vi "Process.vi"(8 "error in":errorcluster, 11 "instrument.PPMS":refnum<class "instrument.PPMS.lvclass">) -> (0 "error out":errorcluster, 3 "instrument.PPMS out":refnum<class "instrument.PPMS.lvclass">)   [LabVIEW 2019, in "instrument.PPMS.lvclass"]
doc: "---------------------------------------------------------------\nJKI State Machine Objects™\nhttp://jki.net/state-machine-objects/\nCopyright (C) 2005-2015, JKI <info@jki.net>\nALL RIGHTS RESERVED"
uses:
  instrument.PPMS.lvclass
  <vilib>/JKI/JKI SMO/SMO/SMO.lvclass
  <userlib>/LevyLab/Instrument Framework/Instrument Types/Cryostat/Instrument.Cryostat.lvclass
  <userlib>/LevyLab/RemoteControl/RemoteControl/Typedefs/Message--Cluster.ctl
  <userlib>/LevyLab/RemoteControl/RemoteControl/RemoteControl.lvclass
  Typedefs/Private Events--MessageToProcess.ctl
  <userlib>/LevyLab/Instrument Framework/Instrument/Instrument.lvclass
  <userlib>/LevyLab/Debug/Debug.lvlib
  C:/Program Files (x86)/National Instruments/LabVIEW 2019/user.lib/LevyLab/Instrument Framework/Instrument Types/Cryostat/Instrument.Cryostat.lvclass
  C:/Program Files (x86)/National Instruments/LabVIEW 2019/user.lib/LevyLab/Instrument Framework/Instrument/Instrument.lvclass
  C:/Program Files (x86)/National Instruments/LabVIEW 2019/vi.lib/JKI/JKI SMO/SMO/SMO.lvclass
panel:
  out "Log Address":string
  out "Log Data":variant
  out "Commands":string
  out "Status":string
  in  "STOP":bool
  # "PPMS Monitor"
  # "THIS ONE IS NOT THE UI"
  # "For instructions on how to use the JKI State Machine Objects, examples and video tutorials, visit:\nhttp://jki.net/state-machine-objects/\n\nJKI State Machine Objects™\nhttp://jki.net/state-machine-objects/\nCopyright (C) 2005-2015, JKI <info@jki.net>\nALL RIGHTS RESERVED"
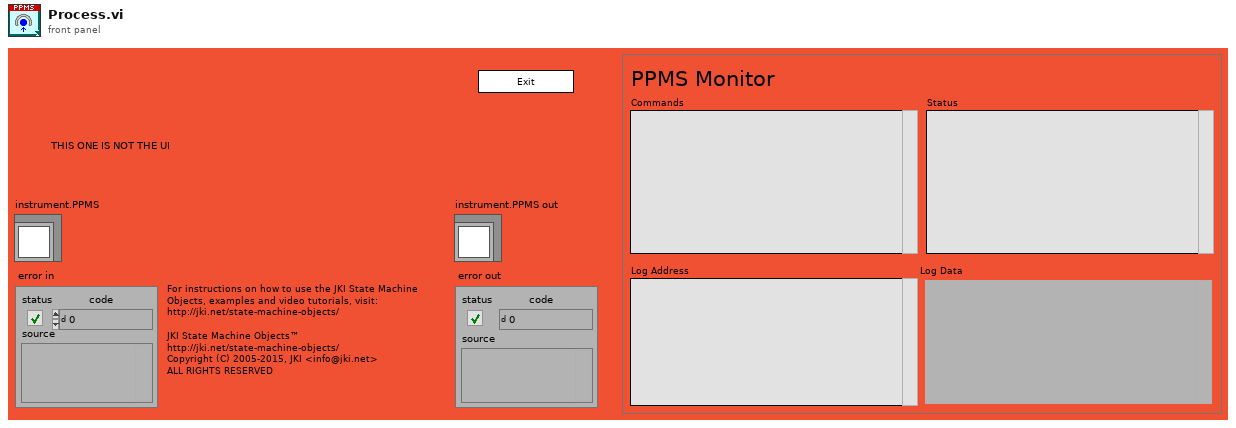
[diagram p1: front panel]
types:
  T1 = enum32{"invalid app kind", "Development System", "Run Time System", "Student Edition", "Embedded LabVIEW", "Evaluation", "Custom"}
  T2 = enum32{"Invalid", "Standard", "Closed", "Hidden", "Minimized", "Maximized"}
  T3 = typedef "RemoteControl.lvlib/RemoteControl.lvclass/Message--Cluster.ctl" = cluster{"Command":string, "Data":variant, "ID":string, "error":errorcluster}
  T4 = typedef "instrument.PPMS.lvclass/Private Events--MessageToProcess.ctl" = cluster{"Message":T3}
  T5 = cluster{"Core":cluster{"Current VI Reference":refnum<vi>, "Close Panel on Exit?":bool, "Last Error":cluster{"error":errorcluster, "previous state":string, "remaining states":string}, "Shutdown?":bool}, "SMO":refnum<class "instrument.PPMS.lvclass">, "MessageToProcess":T4}
  T6 = cluster{"Current VI Reference":refnum<vi>, "Close Panel on Exit?":bool, "Last Error":cluster{"error":errorcluster, "previous state":string, "remaining states":string}, "Shutdown?":bool}
  T7 = typedef "instrument.PPMS.lvclass/PPMS.getAll--cluster.ctl" = cluster{"Chamber Status":string, "Helium Level":dbl, "Temperature":dbl, "Temperature Status":string, "Magnetic Field":dbl, "Magnet Status":string, "Position":dbl}
  T8 = typedef "Debug.lvlib/Attribute.Debug.lvclass/DebugBehavior.ctl" = enum16{"Normal", "Debug"}
  T9 = typedef "SMO.lvclass/Protected Events.ctl" = cluster{"StopProcesses":refnum<user-event>, "AbortProcesses":refnum<user-event>, "Config Changed":refnum<user-event>, "Dependency":refnum<user-event>}
  T10 = typedef "instrument.PPMS.lvclass/Private Events--Cluster.ctl" = cluster{"MessageToProcess":refnum<user-event>}
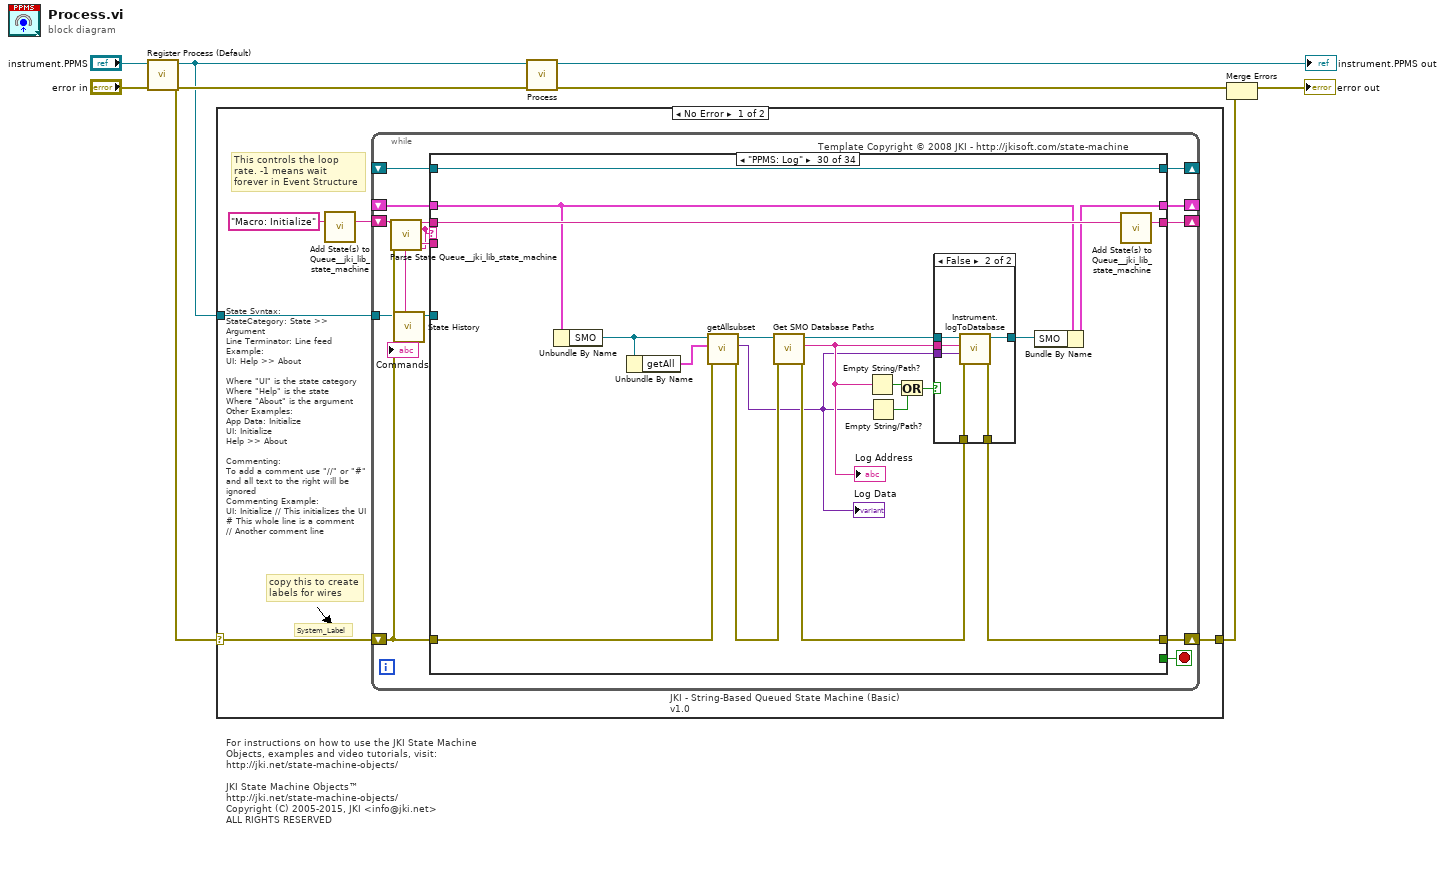
[diagram p0: block diagram]
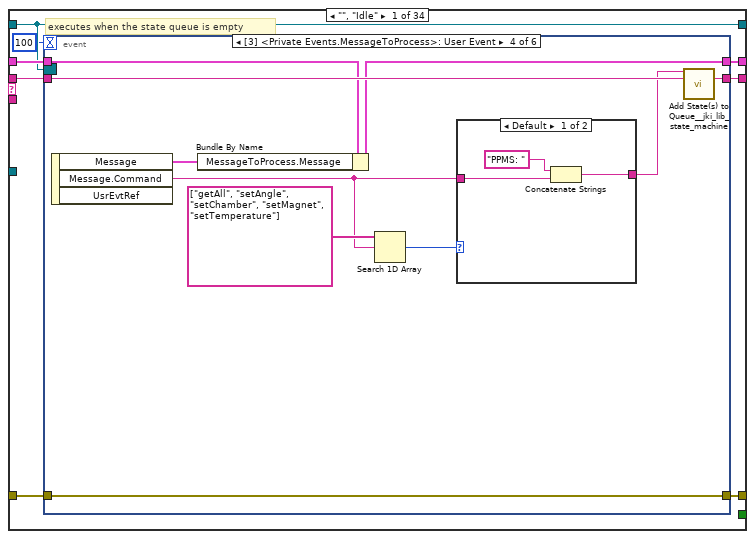
[diagram p2: hidden frame]
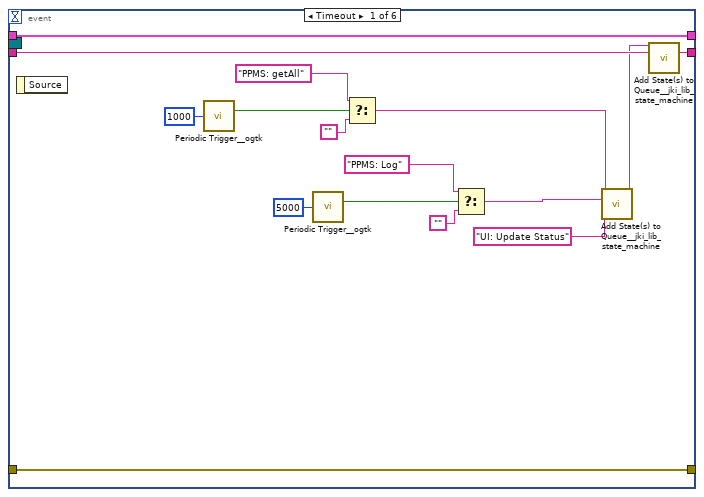
[diagram p3: hidden frame]
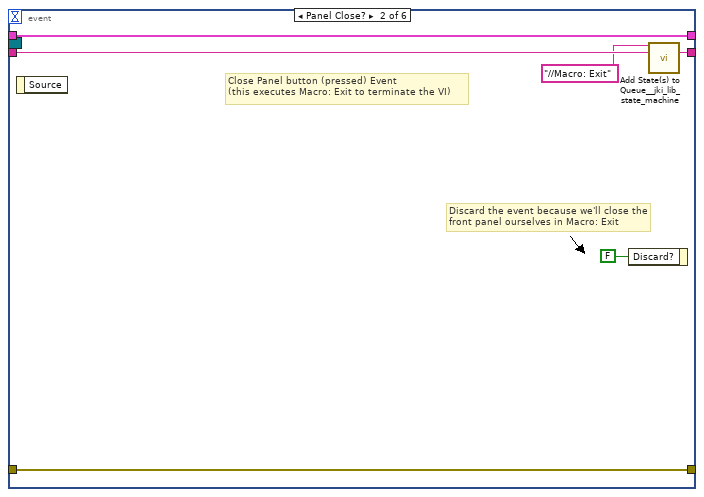
[diagram p4: hidden frame]
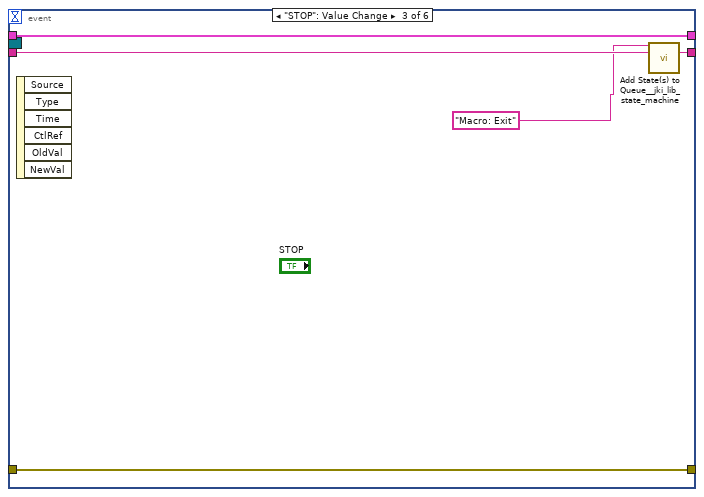
[diagram p5: hidden frame]
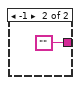
[diagram p6: hidden frame]
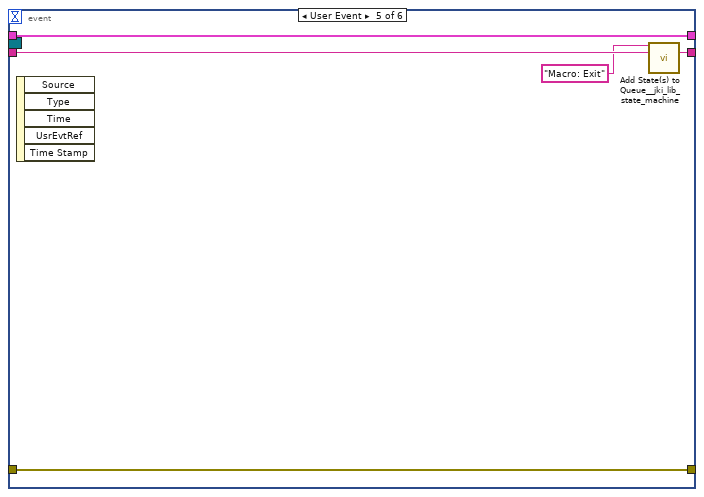
[diagram p7: hidden frame]
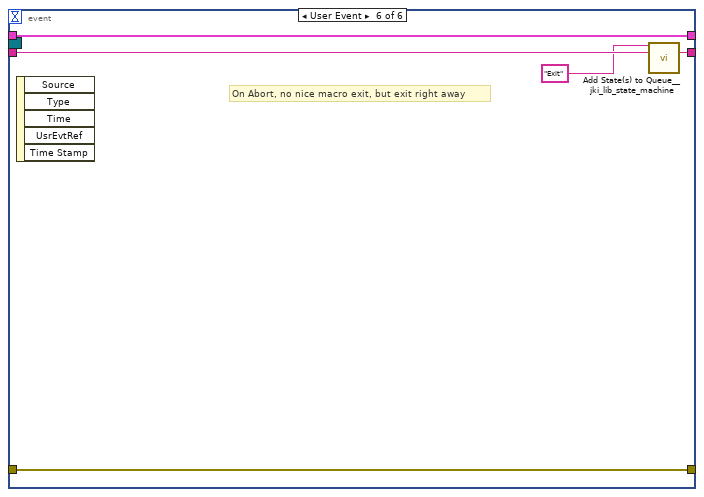
[diagram p8: hidden frame]
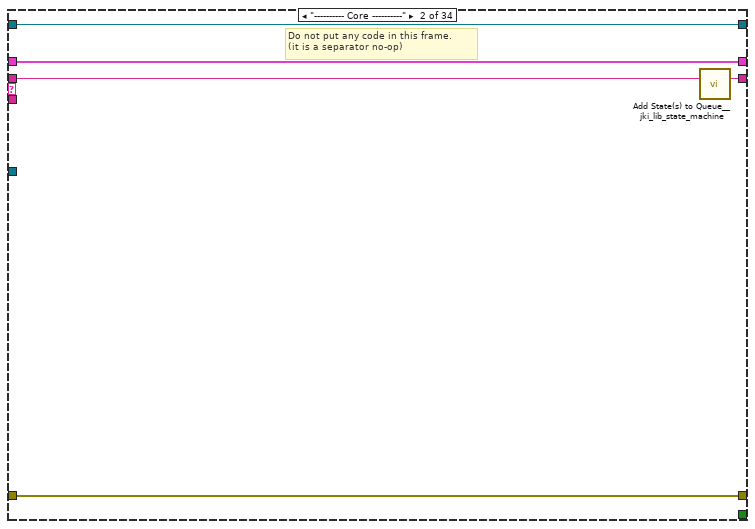
[diagram p9: hidden frame]
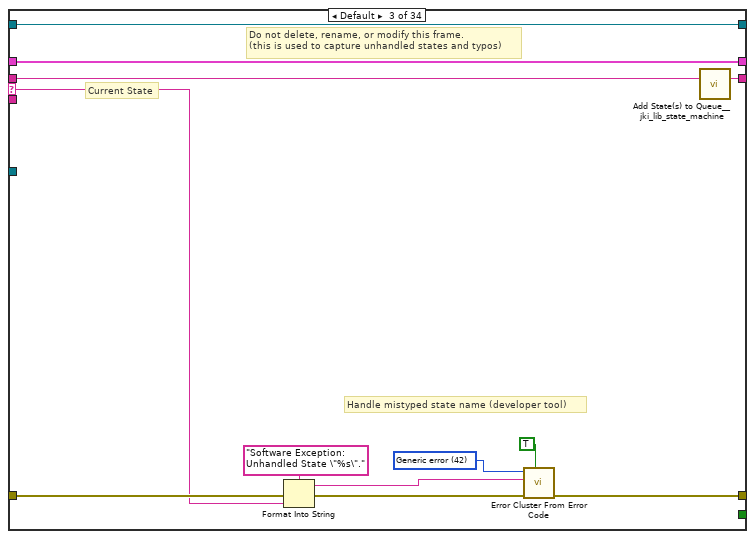
[diagram p10: hidden frame]
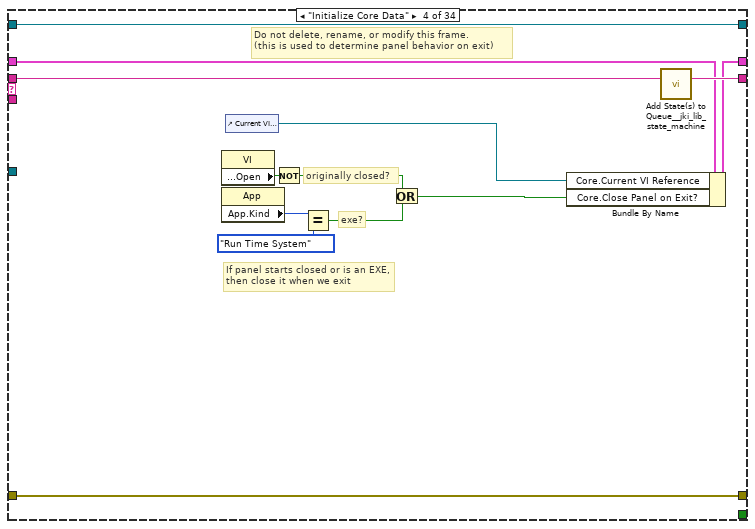
[diagram p11: hidden frame]
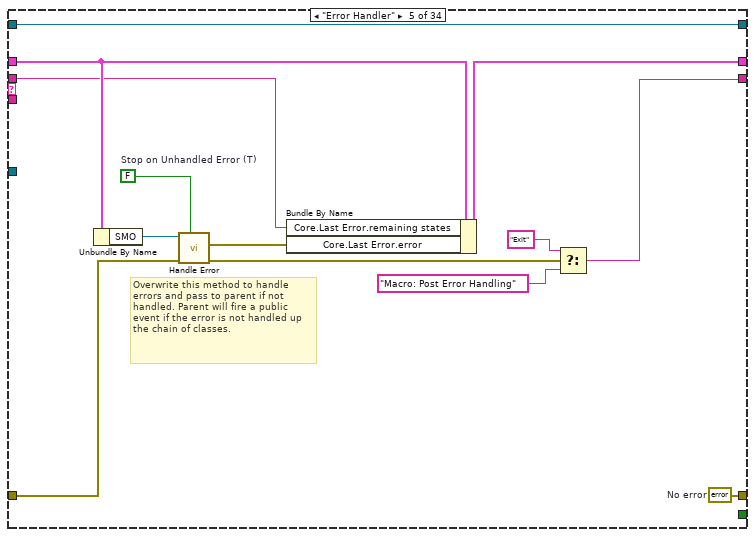
[diagram p12: hidden frame]
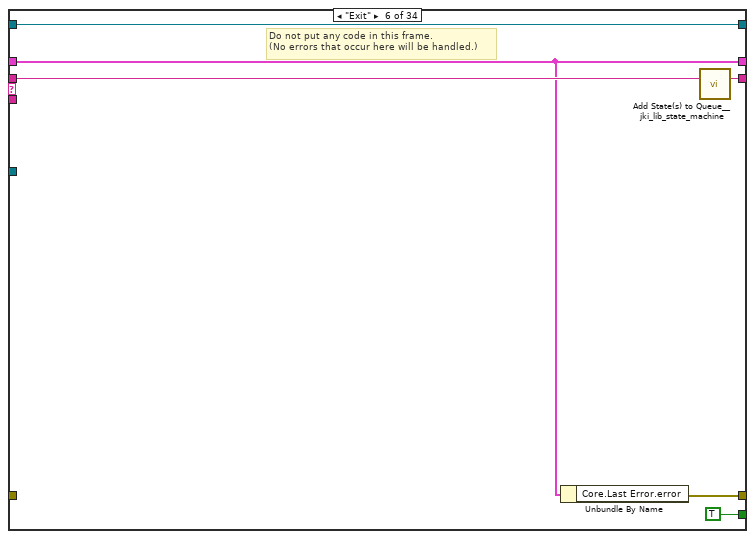
[diagram p13: hidden frame]
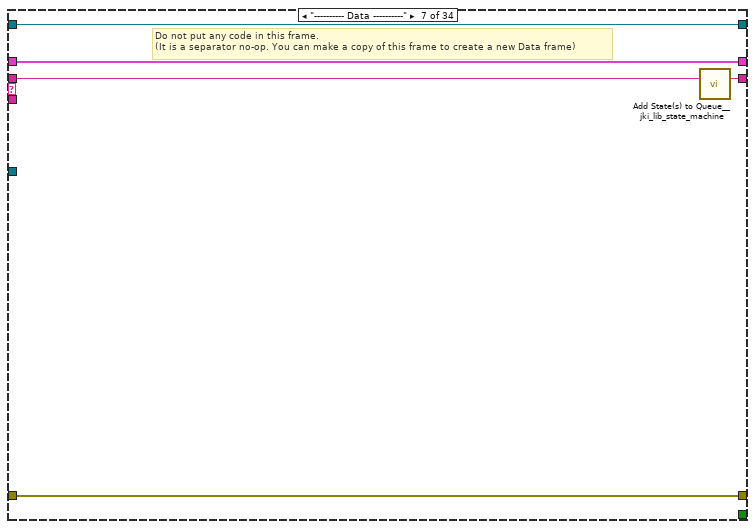
[diagram p14: hidden frame]
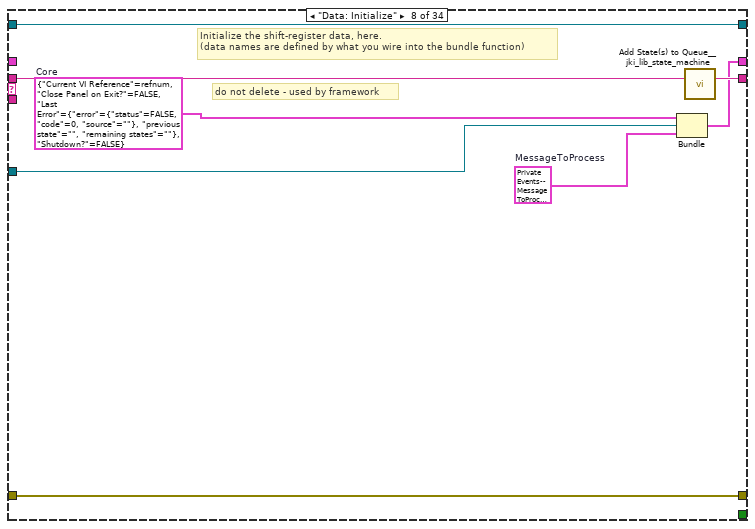
[diagram p15: hidden frame]
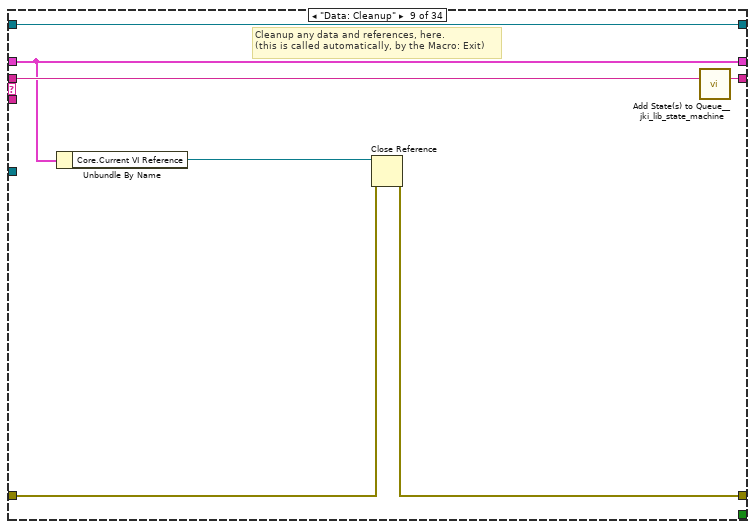
[diagram p16: hidden frame]
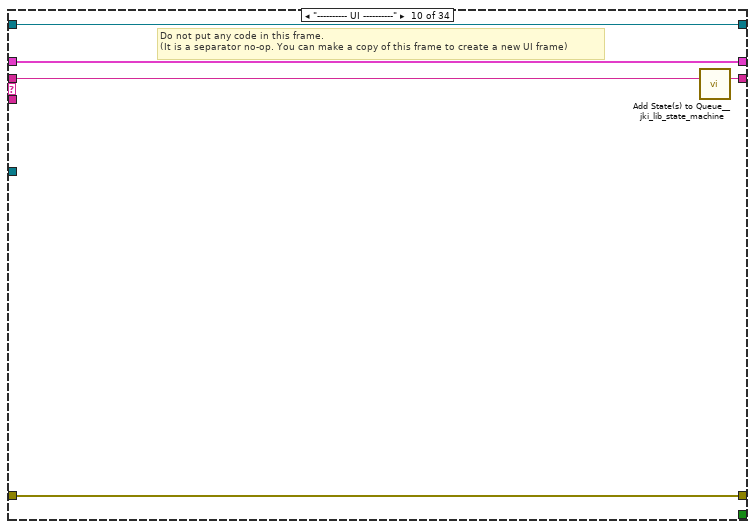
[diagram p17: hidden frame]
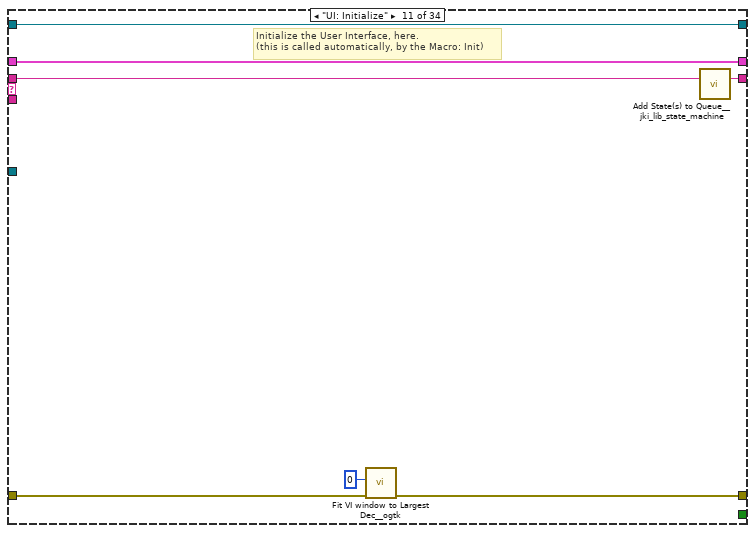
[diagram p18: hidden frame]
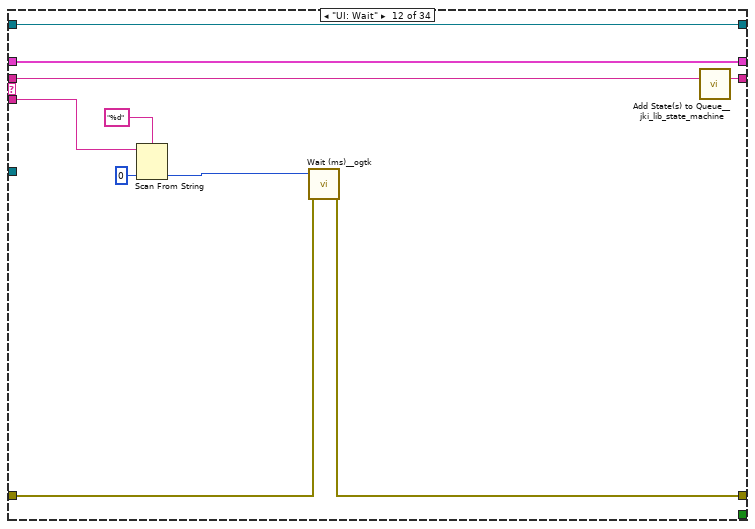
[diagram p19: hidden frame]
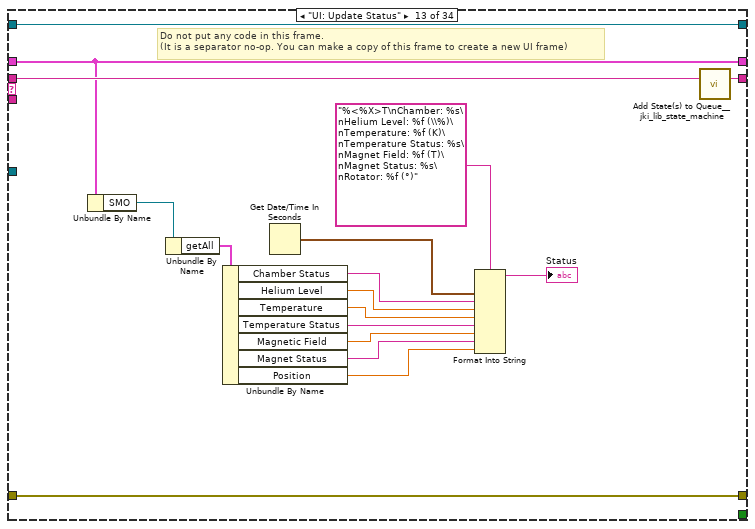
[diagram p20: hidden frame]
diagram:
  # "For instructions on how to use the JKI State Machine Objects, examples and video tutorials, visit:\nhttp://jki.net/state-machine-objects/\n\nJKI State Machine Objects™\nhttp://jki.net/state-machine-objects/\nCopyright (C) 2005-2015, JKI <info@jki.net>\nALL RIGHTS RESERVED"
  n1 = call <vilib>:"Register Process (Default).vi"("error in (no error)"="error in", "SMO"="instrument.PPMS") -> ("error out"=w5:errorcluster, "SelfRef"=w4:refnum<class "instrument.PPMS.lvclass">)  [unwired: 8 in]
  n2 = case shown="No Error" w5 {
    selector: w5 -> [w10 w454]
    tunnel: w4 -> [w11 _]
    tunnel: [w9 w454] -> w1
    frame No Error {
      # "State Syntax:\nStateCategory: State >> Argument\nLine Terminator: Line feed\nExample:\nUI: Help >> About\n\nWhere \"UI\" is the state category\nWhere \"Help\" is the state\nWhere \"About\" is the argument\nOther Examples:\nApp Data: Initialize\nUI: Initialize\nHelp >> About\n\nCommenting:\nTo add a comment use \"//\" or \"#\" and all text to the right will be ignored\nCommenting Example:\nUI: Initialize // This initializes the UI\n# This whole line is a comment\n// Another comment line"
      # "copy this to create labels for wires"
      # "This controls the loop rate. -1 means wait forever in Event Structure"
      # "System_Label"
      n3 = call <vilib>:"Add State(s) to Queue__jki_lib_state_machine.vi"("State(s) in (\"\")"="Macro: Initialize") -> ("States Out"=w13:string)  [unwired: 14 in]
      n4 = while "JKI - String-Based Queued State Machine (Basic) v1.0" {
        shift-right: [w23] -> _
        shift-left: _ -> [w19]
        shift-right: [w26] -> w9
        shift-left: w10 -> [w22]
        shift-right: [w25] -> _
        shift-left: w13 -> [w27]
        tunnel: w11 -> [w14]
        shift-right: [w21] -> _
        shift-left: _ -> [w20]
        stop <- w24 stop-if-true
        # "Template Copyright © 2008 JKI - http://jkisoft.com/state-machine"
        n5 = call <vilib>:"Parse State Queue__jki_lib_state_machine.vi"("State Queue"=w27, "Error In (no error)"=w22) -> ("Remaining States"=w28:string, "Current State"=w17:string, "Arguments"=w18:string)  [unwired: 11 in]
        n6 = call <userlib>:"State History.vi"("Current State"=w17, "SMO"=w14) -> ("SMO"=w15:refnum<class "instrument.PPMS.lvclass">, "History"=→"Commands":string)  [unwired: 8 in]
        n7 = case shown="\"PPMS: Log\"" w17 {
          selector: w17 -> [_ _ w94 _ _ _ _ _ _ _ _ _ _ _ _ _ _ _ _ _ _ _ _ _ _ _ _ _ _ _ _ _ _ _]
          tunnel: w28 -> [w36 w92 w98 w117 w118 w136 w141 w149 w156 w161 w168 w178 w195 w202 w218 w250 w259 w273 w290 w311 w316 w327 w332 w345 w351 w356 w365 w374 w386 w405 w423 w433 w443 w453]
          tunnel: w18 -> [_ _ _ _ _ _ _ _ _ _ _ w170 _ w196 w212 _ _ _ _ _ _ _ _ _ _ _ _ _ _ _ _ _ _ _]
          tunnel: w19 -> [w34 w89 w96 w108 w126 w132 w138 _ w152 w158 w166 w175 w182 w200 w214 w247 w255 w261 w280 w295 w313 w324 w329 w343 w349 w353 w361 w370 w380 w400 w419 w429 w439 w449]
          tunnel: [w33 w90 w100 w114 w127 w131 w139 w142 w153 w159 w163 w174 w193 w197 w215 w248 w257 w271 w288 w309 w314 w318 w330 w338 w347 w354 w358 w366 w377 w399 w415 w425 w435 w445] -> w26
          tunnel: w22 -> [w32 w90 w99 w114 w128 _ w139 w142 w150 w159 w162 w173 w193 w198 w216 w248 w257 w271 w288 w309 w314 w319 w330 w339 w347 w354 w359 w367 w382 w392 w416 w426 w436 w446]
          tunnel: [w35 w91 w97 w116 w119 w135 w140 w148 w155 w160 w167 w177 w194 w201 w217 w249 w258 w272 w289 w310 w315 w326 w331 w344 w350 w355 w364 w373 w385 w404 w422 w432 w442 w452] -> w25
          tunnel: [_ _ _ _ _ TRUE _ _ _ _ _ _ _ _ _ _ _ _ _ _ _ _ _ _ _ _ _ _ _ _ _ _ _ _] -> w24
          tunnel: [w31 w89 w96 w115 w125 w132 w138 w146 w152 w158 w166 w175 w182 w200 w214 w247 w255 w262 w281 w296 w313 w324 w329 w343 w349 w353 w362 w371 w381 w401 w420 w430 w440 w450] -> w23
          tunnel: w15 -> [_ _ _ _ _ _ _ w143 _ _ _ _ _ _ _ _ _ _ _ _ _ _ _ _ _ _ _ _ _ _ _ _ _ _]
          tunnel: [w30 w88 w93 w105 w130 w133 w137 w147 w151 w157 w165 w176 w192 w199 w211 w246 w256 w270 w287 w303 w312 w325 w328 w342 w348 w352 w363 w372 w384 w403 w421 w431 w441 w451] -> w21
          tunnel: w20 -> [w30 w88 w93 w105 w130 w133 w137 w147 w151 w157 w165 w176 w192 w199 w211 w246 w256 w270 w287 w303 w312 w325 w328 _ w348 w352 w363 w372 w384 w403 w421 w431 w441 w451]
          frame "", "Idle" {
            # "executes when the state queue is empty"
            n8 = event shown="[3] <Private Events.MessageToProcess>: User Event" {
              selector: w30 -> [_ _ _ _ _ _]
              dyn-events: _ -> [_ _ _ _ _ _]
              timeout: 100 -> [_ _ _ _ _ _]
              tunnel: w36 -> [w52 w58 w63 w73 w82 w87]
              tunnel: [w51 w57 w62 w72 w81 w86] -> w35
              tunnel: w34 -> [w50 w55 w60 w68 w79 w84]
              tunnel: [w49 w56 w61 w71 w80 w85] -> w33
              tunnel: w32 -> [w49 w56 w61 w71 w80 w85]
              tunnel: [w50 w55 w60 w69 w79 w84] -> w31
              event Timeout {
                n9 = event-data() -> ()  [unwired: 1 in, 1 out]
                n10 = call <userlib>:"Periodic Trigger__ogtk.vi"("time (ms)"=u32 1000) -> ("Triggered"=w48:bool)  [unwired: 12 in, 2 out]
                n11 = call <userlib>:"Periodic Trigger__ogtk.vi"("time (ms)"=u32 5000) -> ("Triggered"=w39:bool)  [unwired: 12 in, 2 out]
                n12 = Select(t="PPMS: getAll", s=w48, f="") -> (s? t:f=w43:string)
                n13 = Select(t="PPMS: Log", s=w39, f="") -> (s? t:f=w37:string)
                n14 = call <vilib>:"Add State(s) to Queue__jki_lib_state_machine.vi"("State(s) in Front (\"\")"=w43, "State(s) in (\"\")"=w37, "State(s) at Back (\"\")"="UI: Update Status") -> ("States Out"=w42:string)  [unwired: 12 in]
                n15 = call <vilib>:"Add State(s) to Queue__jki_lib_state_machine.vi"("State(s) in Front (\"\")"=w42, "State(s) in (\"\")"=w52) -> ("States Out"=w51:string)  [unwired: 13 in]
              }
              event Panel Close? {
                # "Discard the event because we'll close the front panel ourselves in Macro: Exit"
                # "Close Panel button (pressed) Event\n(this executes Macro: Exit to terminate the VI)"
                n16 = event-data() -> ()  [unwired: 1 in, 1 out]
                n17 = event-data("Discard?"=FALSE) -> ()  [unwired: 1 in, 1 out]
                n18 = call <vilib>:"Add State(s) to Queue__jki_lib_state_machine.vi"("State(s) in Front (\"\")"="//Macro: Exit", "State(s) in (\"\")"=w58) -> ("States Out"=w57:string)  [unwired: 13 in]
              }
              event "STOP": Value Change {
                n19 = event-data() -> ()  [unwired: 1 in, 6 out]
                n20 = call <vilib>:"Add State(s) to Queue__jki_lib_state_machine.vi"("State(s) in Front (\"\")"="Macro: Exit", "State(s) in (\"\")"=w63) -> ("States Out"=w62:string)  [unwired: 13 in]
              }
              event User Event {
                n21 = event-data() -> ("Message"=w70:T3, "Message.Command"=w64:string)  [unwired: 1 in, 1 out]
                n22 = Bundle By Name(cluster=w68, "MessageToProcess.Message"=w70) -> (w69:T5)
                n23 = Search 1D Array(1D array=string[] ["getAll", "setAngle", "setChamber", "setMagnet", "setTemperature"], element=w64) -> (index of element=w67:i32)  [unwired: 1 in]
                n24 = case shown="Default" w67 {
                  tunnel: [w76 ""] -> w66
                  tunnel: w64 -> [w75 _]
                  frame Default {
                    n25 = Concatenate Strings("PPMS: ", w75) -> (w76:string)
                  }
                  frame -1 {
                  }
                }
                n26 = call <vilib>:"Add State(s) to Queue__jki_lib_state_machine.vi"("State(s) in Front (\"\")"=w66, "State(s) in (\"\")"=w73) -> ("States Out"=w72:string)  [unwired: 13 in]
              }
              event User Event {
                n27 = event-data() -> ()  [unwired: 1 in, 5 out]
                n28 = call <vilib>:"Add State(s) to Queue__jki_lib_state_machine.vi"("State(s) in Front (\"\")"="Macro: Exit", "State(s) in (\"\")"=w82) -> ("States Out"=w81:string)  [unwired: 13 in]
              }
              event User Event {
                # "On Abort, no nice macro exit, but exit right away"
                n29 = event-data() -> ()  [unwired: 1 in, 5 out]
                n30 = call <vilib>:"Add State(s) to Queue__jki_lib_state_machine.vi"("State(s) in Front (\"\")"="Exit", "State(s) in (\"\")"=w87) -> ("States Out"=w86:string)  [unwired: 13 in]
              }
            }
          }
          frame "---------- Core ----------" {
            # "Do not put any code in this frame.\n(it is a separator no-op)"
            n31 = call <vilib>:"Add State(s) to Queue__jki_lib_state_machine.vi"("State(s) in (\"\")"=w92) -> ("States Out"=w91:string)  [unwired: 14 in]
          }
          frame Default {
            w103 = 42 items=["No error", "Argument error", "Memory is full", "Out of zone", "End of file", "File already open", "Generic file I/O error", "File not found", "File permission error", "Disk is full", "Duplicate path", "Too many files open", "System feature not enabled", "Resource file not found", "Cannot add resource", "Resource not found", "Image not found", "Image memory error", "Pen does not exist", "Config type invalid", "Config token not found", "Config parse error", "Config memory error", "Bad external code format", "Bad external code offset", "External code not present", "Null window", "Destroy window error", "Null menu", "Print aborted", "Bad print record", "Print driver error", "Windows error during printing", "Memory error during printing", "Print dialog error", "Generic print error", "Invalid device refnum", "Device not found", "Device parameter error", "Device unit error", "Cannot open device", "Device call aborted", "Generic error", "Cancelled by user", "Object ID too low", "Object ID too high", "Object not in heap", "Unknown heap", "Unknown object (invalid DefProc)", "Unknown object (DefProc not in table)", "Message out of range", "Invalid (null) method", "Unknown message", "Manager call not supported", "Bad address", "Network operation in progress", "Network operation timed out", "Connection is busy", "Network attribute not supported", "Network error", "Address in use", "System out of memory", "Connection aborted", "Connection refused", "Not connected", "Already connected", "Connection closed", "Initialization error (interapplication manager)", "Bad occurrence", "Wait on unbound occurrence handler", "Occurrence queue overflow", "Datalog type conflict", "Unused", "Unrecognized type (interapplication manager)", "Memory corrupt", "Failed to make temporary DLL", "Old CIN version", "Drag socket not found", "Failed to load drop-object", "Failed to register OLE object", "Failed to release OLE object", "Format specifier type mismatch", "Unknown format specifier", "Too few format specifiers", "Too many format specifiers", "Scan failed", "Newer CIN version", "Error converting to variant", "Runtime menu error", "Password tampered", "Variant attribute not found", "Incompatible variant data type", "Event data is not available", "Event Store is not present", "Occurrence is not found", "Event Queue is not created", "Event info is not available", "Refnum passed is NULL", "Error retrieving Class GUID", "Error retrieving CoClass GUID", "Error retrieving TypeLib GUID.", "Bad built application magic bytes.", "Specific driver is different from the specific driver associated with the Logical Name.", "There is no session opened to the class driver.", "Max Error", "MAX - Error with config objects", "MAX - Error loading configuration", "MAX - Group not supported"]
            # "Current State"
            # "Do not delete, rename, or modify this frame.\n(this is used to capture unhandled states and typos)"
            # "Handle mistyped state name (developer tool)"
            n32 = Format Into String(format string="Software Exception: Unhandled State \"%s\"." ("message"), error in=w99, w94) -> (resulting string=w102:string, error out=w101:errorcluster)  [unwired: 1 in]
            n33 = call <vilib>:"Error Cluster From Error Code.vi"("show call chain? (False)"=TRUE, "error in (no error)"=w101, "error message (\"\")"=w102, "error code (0)"=w103) -> ("error out"=w100:errorcluster)  [unwired: 5 in]
            n34 = call <vilib>:"Add State(s) to Queue__jki_lib_state_machine.vi"("State(s) in (\"\")"=w98) -> ("States Out"=w97:string)  [unwired: 14 in]
          }
          frame "Initialize Core Data" {
            # "Do not delete, rename, or modify this frame.\n(this is used to determine panel behavior on exit)"
            # "originally closed?"
            # "exe?"
            # "If panel starts closed or is an EXE, then close it when we exit"
            n35 = property class="VI"() -> ("Front Panel.Open"=w113:bool)  [unwired: 2 in, 2 out]
            n36 = property class="App"() -> ("App.Kind"=w112:T1)  [unwired: 2 in, 2 out]
            n37 = control-ref of="Current VI Reference"() -> (w106:refnum<vi>)
            n38 = Not(x=w113) -> (.not. x?=w110:bool)
            n39 = Equal?(x=w112, y=T1."Run Time System" ("Application:Kind")) -> (x = y?=w109:bool)
            n40 = Or(x=w110, y=w109) -> (x .or. y?=w107:bool)
            n41 = Bundle By Name(cluster=w108, "Core.Current VI Reference"=w106, "Core.Close Panel on Exit?"=w107) -> (w115:T5)
            n42 = call <vilib>:"Add State(s) to Queue__jki_lib_state_machine.vi"("State(s) in (\"\")"=w117) -> ("States Out"=w116:string)  [unwired: 14 in]
          }
          frame "Error Handler" {
            w121 = FALSE  # Stop on Unhandled Error (T)
            w127 = errorcluster {"status"=FALSE, "code"=0, "source"=""}  # No error
            # "Overwrite this method to handle errors and pass to parent if not handled. Parent will fire a public event if the error is not handled up the chain of classes."
            n43 = Unbundle By Name(w126) -> ("SMO"=w129:refnum<class "instrument.PPMS.lvclass">)
            n44 = call-dynamic "Handle Error.vi"("Stop on Unhandled Error (T)"=w121, "error in"=w128, "SMO"=w129) -> ("handling error"=w122:errorcluster, "Unhandled error"=w124:errorcluster)  [unwired: 6 in, 1 out]
            n45 = Bundle By Name(cluster=w126, "Core.Last Error.remaining states"=w118, "Core.Last Error.error"=w124) -> (w125:T5)
            n46 = Select(t="Exit", s=w122, f="Macro: Post Error Handling") -> (s? t:f=w119:string)
          }
          frame "Exit" {
            # "Do not put any code in this frame.\n(No errors that occur here will be handled.)"
            n47 = Unbundle By Name(w132) -> ("Core.Last Error.error"=w131:errorcluster)
            n48 = call <vilib>:"Add State(s) to Queue__jki_lib_state_machine.vi"("State(s) in (\"\")"=w136) -> ("States Out"=w135:string)  [unwired: 14 in]
          }
          frame "---------- Data ----------" {
            # "Do not put any code in this frame.\n(It is a separator no-op. You can make a copy of this frame to create a new Data frame)"
            n49 = call <vilib>:"Add State(s) to Queue__jki_lib_state_machine.vi"("State(s) in (\"\")"=w141) -> ("States Out"=w140:string)  [unwired: 14 in]
          }
          frame "Data: Initialize" {
            w144 = T6 {"Current VI Reference"=refnum, "Close Panel on Exit?"=FALSE, "Last Error"={"error"={"status"=FALSE, "code"=0, "source"=""}, "previous state"="", "remaining states"=""}, "Shutdown?"=FALSE}  # Core
            w145 = T4 {"Message"={"Command"="", "Data"=variant(string ""), "ID"="", "error"={"status"=FALSE, "code"=0, "source"=""}}}  # MessageToProcess
            # "do not delete - used by framework"
            # "Initialize the shift-register data, here.\n(data names are defined by what you wire into the bundle function)"
            n50 = Bundle("Core"=w144, "SMO"=w143, "MessageToProcess"=w145) -> (w146:T5)  [unwired: 1 in]
            n51 = call <vilib>:"Add State(s) to Queue__jki_lib_state_machine.vi"("State(s) in (\"\")"=w149) -> ("States Out"=w148:string)  [unwired: 14 in]
          }
          frame "Data: Cleanup" {
            # "Cleanup any data and references, here.\n(this is called automatically, by the Macro: Exit)"
            n52 = Unbundle By Name(w152) -> ("Core.Current VI Reference"=w154:refnum<vi>)
            n53 = Close Reference(reference=w154, error in (no error)=w150) -> (error out=w153:errorcluster)
            n54 = call <vilib>:"Add State(s) to Queue__jki_lib_state_machine.vi"("State(s) in (\"\")"=w156) -> ("States Out"=w155:string)  [unwired: 14 in]
          }
          frame "---------- UI ----------" {
            # "Do not put any code in this frame.\n(It is a separator no-op. You can make a copy of this frame to create a new UI frame)"
            n55 = call <vilib>:"Add State(s) to Queue__jki_lib_state_machine.vi"("State(s) in (\"\")"=w161) -> ("States Out"=w160:string)  [unwired: 14 in]
          }
          frame "UI: Initialize" {
            # "Initialize the User Interface, here.\n(this is called automatically, by the Macro: Init)"
            n56 = call <userlib>:"Fit VI window to Largest Dec__ogtk.vi"("error in (no error)"=w162, "border spacing (2 px)"=0) -> ("error out"=w163:errorcluster)  [unwired: 4 in, 1 out]
            n57 = call <vilib>:"Add State(s) to Queue__jki_lib_state_machine.vi"("State(s) in (\"\")"=w168) -> ("States Out"=w167:string)  [unwired: 14 in]
          }
          frame "UI: Wait" {
            n58 = Scan From String(format string="%d", input string=w170, default 1=u32 0 ("default value 1")) -> (output 1=w169:u32)  [unwired: 2 in, 3 out]
            n59 = call <userlib>:"Wait (ms)__ogtk.vi"("error in (no error)"=w173, "milliseconds to wait"=w169) -> ("error out"=w174:errorcluster)  [unwired: 8 in, 1 out]
            n60 = call <vilib>:"Add State(s) to Queue__jki_lib_state_machine.vi"("State(s) in (\"\")"=w178) -> ("States Out"=w177:string)  [unwired: 14 in]
          }
          frame "UI: Update Status" {
            # "Do not put any code in this frame.\n(It is a separator no-op. You can make a copy of this frame to create a new UI frame)"
            n61 = Unbundle By Name(w182) -> ("SMO"=w180:refnum<class "instrument.PPMS.lvclass">)
            n62 = Unbundle By Name(w180) -> ("getAll"=w181:T7)
            n63 = Unbundle By Name(w181) -> ("Chamber Status"=w190:string, "Helium Level"=w189:dbl, "Temperature"=w188:dbl, "Temperature Status"=w187:string, "Magnetic Field"=w186:dbl, "Magnet Status"=w185:string, "Position"=w184:dbl)
            n64 = Get Date/Time In Seconds() -> (seconds since 1Jan1904=w179:timestamp)
            n65 = Format Into String(format string="%<%X>T\nChamber: %s\nHelium Level: %f (\\%)\nTemperature: %f (K)\nTemperature Status: %s\nMagnet Field: %f (T)\nMagnet Status: %s\nRotator: %f (°)", w179, w190, w189, w188, w187, w186, w185, w184) -> (resulting string=→"Status":string)  [unwired: 2 in, 1 out]
            n66 = call <vilib>:"Add State(s) to Queue__jki_lib_state_machine.vi"("State(s) in (\"\")"=w195) -> ("States Out"=w194:string)  [unwired: 14 in]
          }
          frame "UI: Cursor Set" {
            # "Argument"
            # "Initialize the User Interface, here.\n(this is called automatically, by the Macro: Init)"
            n67 = disable-structure shown="Default" {
              disable-tunnel: w198 -> [w203 w206]
              disable-tunnel: [w203 w205] -> w197
              disable-tunnel: w196 -> [_ w204]
              frame condition #0 {
              }
              frame condition #1 (active) {
                n68 = case shown="\"Idle\", Default" w204 {
                  tunnel: w206 -> [w208 w210]
                  tunnel: [w207 w209] -> w205
                  frame "Idle", Default {
                    n69 = call <vilib>:"Unset Busy.vi"("error in (no error)"=w208) -> ("error out"=w207:errorcluster)  [unwired: 10 in]
                  }
                  frame "Busy" {
                    n70 = call <vilib>:"Set Busy.vi"("error in (no error)"=w210) -> ("error out"=w209:errorcluster)  [unwired: 9 in, 1 out]
                  }
                }
              }
            }
            n71 = call <vilib>:"Add State(s) to Queue__jki_lib_state_machine.vi"("State(s) in (\"\")"=w202) -> ("States Out"=w201:string)  [unwired: 14 in]
          }
          frame "UI: Front Panel State" {
            # "Argument"
            # "Set Front Panel Open or Closed\n(Usage: \"UI: Front Panel State >> Open|Close\")"
            n72 = Unbundle By Name(w214) -> ("Core.Current VI Reference"=w213:refnum<vi>)
            n73 = disable-structure shown="Default" {
              disable-tunnel: w216 -> [w222 w245]
              disable-tunnel: [w221 w245] -> w215
              disable-tunnel: w213 -> [w220 _]
              disable-tunnel: w212 -> [w219 _]
              frame condition #0 (active) {
                n74 = case shown="\"Open\", Default" w219 {
                  tunnel: w222 -> [w226 w239]
                  tunnel: [w228 w240] -> w221
                  tunnel: w220 -> [w227 w237]
                  frame "Open", Default {
                    n75 = property class="VI"(reference=w227, error in=w226) -> (reference out=w224:refnum<vi>, error out=w225:errorcluster, "FP.State"=w223:T2)
                    n76 = case shown="\"Closed\"" w223 {
                      tunnel: [w231 w234] -> w228
                      tunnel: w225 -> [w230 w234]
                      tunnel: w224 -> [w229 _]
                      frame "Closed" {
                        n77 = invoke class="VI" method="FP.Open"(reference=w229, error in=w230, "Activate"=TRUE, "State"=T2."Standard") -> (error out=w231:errorcluster)  [unwired: 1 in, 4 out]
                      }
                      frame Default {
                      }
                    }
                  }
                  frame "Close" {
                    n78 = property class="VI"(reference=w237, error in=w239) -> (reference out=w236:refnum<vi>, error out=w238:errorcluster, "FP.State"=w235:T2)
                    n79 = case shown="\"Invalid\", \"Closed\"" w235 {
                      tunnel: [w241 w244] -> w240
                      tunnel: w238 -> [w241 w243]
                      tunnel: w236 -> [_ w242]
                      frame "Invalid", "Closed" {
                      }
                      frame Default {
                        n80 = invoke class="VI" method="FP.Close"(reference=w242, error in=w243) -> (error out=w244:errorcluster)  [unwired: 1 in, 2 out]
                      }
                    }
                  }
                }
              }
              frame condition #1 {
              }
            }
            n81 = call <vilib>:"Add State(s) to Queue__jki_lib_state_machine.vi"("State(s) in (\"\")"=w218) -> ("States Out"=w217:string)  [unwired: 14 in]
          }
          frame "---------- Macro ----------" {
            # "Do not put any code in this frame.\n(It is a separator no-op. You can make a copy of this frame to create a new Macro frame)"
            n82 = call <vilib>:"Add State(s) to Queue__jki_lib_state_machine.vi"("State(s) in (\"\")"=w250) -> ("States Out"=w249:string)  [unwired: 14 in]
          }
          frame "Macro: Initialize" {
            # "Initialization Macro\n(This is called once, when the VI starts)"
            n83 = call <vilib>:"Add State(s) to Queue__jki_lib_state_machine.vi"("State(s) in Front (\"\")"="Data: Initialize\nInitialize Core Data\nEvents: Register", "State(s) in (\"\")"="Process: Sync", "State(s) at Back (\"\")"="UI: Initialize\nUI: Front Panel State >> Close\nMacro: Debug\nPPMS: Open\nPPMS: getAll") -> ("States Out"=w253:string)  [unwired: 12 in]
            n84 = call <vilib>:"Add State(s) to Queue__jki_lib_state_machine.vi"("State(s) in Front (\"\")"=w253, "State(s) in (\"\")"=w259) -> ("States Out"=w258:string)  [unwired: 13 in]
          }
          frame "Macro: Debug" {
            # "exe?"
            # "If pane is an EXE, then close it when we exit"
            # "Macro: Debug\n(get debug behavior)"
            n85 = Unbundle By Name(w261) -> ("Core.Close Panel on Exit?"=w264:bool, "SMO"=w269:refnum<class "instrument.PPMS.lvclass">)
            n86 = property class="App"() -> ("App.Kind"=w267:T1)  [unwired: 2 in, 2 out]
            n87 = Equal?(x=w267, y=T1."Run Time System" ("Application:Kind")) -> (x = y?=w263:bool)
            n88 = call <userlib>:"Get Debug Mode.vi"("SMO"=w269) -> ("Behavior"=w268:T8)  [unwired: 8 in, 2 out]
            n89 = case shown="\"Debug\"" w268 {
              tunnel: [w274 w276] -> w265
              tunnel: w264 -> [w274 _]
              tunnel: w263 -> [_ w278]
              tunnel: [_ "UI: Front Panel State >> Open\nUI: Wait >> 1000"] -> w260
              frame "Normal", Default {
                # "respect core.close"
              }
              frame "Debug" {
                # "keep panel open\nunless exe"
                n90 = Or(x=w278, y=FALSE) -> (x .or. y?=w276:bool)
              }
            }
            n91 = Bundle By Name(cluster=w261, "Core.Close Panel on Exit?"=w265) -> (w262:T5)
            n92 = call <vilib>:"Add State(s) to Queue__jki_lib_state_machine.vi"("State(s) in Front (\"\")"=w260, "State(s) in (\"\")"=w273) -> ("States Out"=w272:string)  [unwired: 13 in]
          }
          frame "Macro: Post Error Handling" {
            # "Clear Last Error?"
            n93 = Unbundle By Name(w280) -> ("Core.Last Error.remaining states"=w282:string, "Core.Shutdown?"=w283:bool)
            n94 = Unbundle By Name(w280) -> ("Core.Last Error.error"=w286:errorcluster)
            n95 = case shown="False" FALSE {
              tunnel: w286 -> [w294 _]
              tunnel: [w294 _] -> w285
              frame False {
              }
              frame True {
              }
            }
            n96 = case shown="False" w283 {
              tunnel: w282 -> [w291 w293]
              tunnel: [w291 w292] -> w279
              frame False {
                # "These are the remaining states (at the moment the error occured). States can be altered according to business logic."
                # "NOT SHUTTING DOWN"
              }
              frame True {
                # "Developer can decide to alter the states but should be aware that during the shutdown process, there are certain states that must be run for the SMO to properly shut itself (and this process) down. As such, one can add states to perform additional clean-ups, but should append the remaining state to be executed."
                # "SHUTTING DOWN"
                n97 = call <vilib>:"Add State(s) to Queue__jki_lib_state_machine.vi"("State(s) in (\"\")"=w293) -> ("States Out"=w292:string)  [unwired: 14 in]
              }
            }
            n98 = Bundle By Name(cluster=w280, "Core.Last Error.error"=w285) -> (w281:T5)
            n99 = call <vilib>:"Add State(s) to Queue__jki_lib_state_machine.vi"("State(s) in Front (\"\")"=w279, "State(s) in (\"\")"=w290) -> ("States Out"=w289:string)  [unwired: 13 in]
          }
          frame "Macro: Exit" {
            # "Exit Macro\n(This is called once, when the VI exits)"
            n100 = Unbundle By Name(w295) -> ("Core.Close Panel on Exit?"=w308:bool)
            n101 = Bundle By Name(cluster=w295, "Core.Shutdown?"=TRUE) -> (w296:T5)
            n102 = Select(t="UI: Front Panel State >> Close", s=w308, f="") -> (s? t:f=w305:string)
            n103 = call <vilib>:"Add State(s) to Queue__jki_lib_state_machine.vi"("State(s) in Front (\"\")"="Data: Cleanup\nEvents: Unregister", "State(s) in (\"\")"="Process: Sync", "State(s) at Back (\"\")"="Exit") -> ("States Out"=w300:string)  [unwired: 12 in]
            n104 = call <vilib>:"Add State(s) to Queue__jki_lib_state_machine.vi"("State(s) in Front (\"\")"="PPMS: Close" ("State(s) in Front (\"\")"), "State(s) in (\"\")"=w305, "State(s) at Back (\"\")"=w300) -> ("States Out"=w304:string)  [unwired: 12 in]
            n105 = call <vilib>:"Add State(s) to Queue__jki_lib_state_machine.vi"("State(s) in Front (\"\")"=w304, "State(s) in (\"\")"=w311) -> ("States Out"=w310:string)  [unwired: 13 in]
          }
          frame "---------- Process ----------" {
            # "Template Separator\n(You can make a copy of, or modify, this frame)"
            n106 = call <vilib>:"Add State(s) to Queue__jki_lib_state_machine.vi"("State(s) in (\"\")"=w316) -> ("States Out"=w315:string)  [unwired: 14 in]
          }
          frame "Process: Sync" {
            n107 = Unbundle By Name(w324) -> ("SMO"=w320:refnum<class "instrument.PPMS.lvclass">)
            n108 = call <vilib>:"WaitOnProcessSync.vi"("error in (no error)"=w319, "SMO"=w320) -> ("error out"=w318:errorcluster, "Don't run?"=w323:bool)  [unwired: 7 in, 1 out]
            n109 = Select(t="Data: Cleanup\nEvents: Unregister\nExit", s=w323, f="") -> (s? t:f=w317:string)
            n110 = call <vilib>:"Add State(s) to Queue__jki_lib_state_machine.vi"("State(s) in Front (\"\")"=w317, "State(s) in (\"\")"=w327) -> ("States Out"=w326:string)  [unwired: 13 in]
          }
          frame "---------- Events ----------" {
            # "Template Separator\n(You can make a copy of, or modify, this frame)"
            n111 = call <vilib>:"Add State(s) to Queue__jki_lib_state_machine.vi"("State(s) in (\"\")"=w332) -> ("States Out"=w331:string)  [unwired: 14 in]
          }
          frame "Events: Register" {
            # "Expand to add\nmore events"
            n112 = Unbundle By Name(w343) -> ("SMO"=w340:refnum<class "instrument.PPMS.lvclass">)
            n113 = call <vilib>:"GetProtectedEvents.vi"("SMO"=w340) -> ("error out"=w336:errorcluster, "SMO Protected Events"=w341:T9, "SMO out"=w335:refnum<class "instrument.PPMS.lvclass">)  [unwired: 8 in]
            n114 = call "PPMS.GetPrivateEvents.vi"("instrument.PPMS in"=w335) -> ("error out"=w333:errorcluster, "Private Events"=w334:T10)  [unwired: 8 in, 1 out]
            n115 = register-events(w341, w334) -> (reference out=w342:refnum<event-registration>, error out=w337:errorcluster)  [unwired: 2 in]
            n116 = Merge Errors(w333, w339, w337, w336) -> (w338:errorcluster)
            n117 = call <vilib>:"Add State(s) to Queue__jki_lib_state_machine.vi"("State(s) in (\"\")"=w345) -> ("States Out"=w344:string)  [unwired: 14 in]
          }
          frame "Events: Unregister" {
            n118 = Unregister For Events(event registration refnum=w348, error in=w347) -> (error out=w346:errorcluster)
            n119 = call <vilib>:"Clear Errors.vi"("error in (no error)"=w346) -> ()  [unwired: 5 in, 2 out]
            n120 = call <vilib>:"Add State(s) to Queue__jki_lib_state_machine.vi"("State(s) in (\"\")"=w351) -> ("States Out"=w350:string)  [unwired: 14 in]
          }
          frame "---------- PPMS ----------" {
            # "Template Separator\n(You can make a copy of, or modify, this frame)"
            n121 = call <vilib>:"Add State(s) to Queue__jki_lib_state_machine.vi"("State(s) in (\"\")"=w356) -> ("States Out"=w355:string)  [unwired: 14 in]
          }
          frame "PPMS: Open" {
            n122 = Unbundle By Name(w361) -> ("SMO"=w357:refnum<class "instrument.PPMS.lvclass">)
            n123 = call-dynamic "Open Hardware.vi"("error in (no error)"=w359, "instrument.PPMS"=w357) -> ("error out"=w358:errorcluster, "instrument.PPMS out"=w360:refnum<class "instrument.PPMS.lvclass">)  [unwired: 8 in]
            n124 = Bundle By Name(cluster=w361, "SMO"=w360) -> (w362:T5)
            n125 = call <vilib>:"Add State(s) to Queue__jki_lib_state_machine.vi"("State(s) in (\"\")"=w365) -> ("States Out"=w364:string)  [unwired: 14 in]
          }
          frame "PPMS: Close" {
            n126 = Unbundle By Name(w370) -> ("SMO"=w369:refnum<class "instrument.PPMS.lvclass">)
            n127 = call-dynamic "Close Hardware.vi"("error in (no error)"=w367, "instrument.PPMS"=w369) -> ("error out"=w366:errorcluster, "instrument.PPMS out"=w368:refnum<class "instrument.PPMS.lvclass">)  [unwired: 8 in]
            n128 = Bundle By Name(cluster=w370, "SMO"=w368) -> (w371:T5)
            n129 = call <vilib>:"Add State(s) to Queue__jki_lib_state_machine.vi"("State(s) in (\"\")"=w374) -> ("States Out"=w373:string)  [unwired: 14 in]
          }
          frame "PPMS: getAll" {
            n130 = Unbundle By Name(w380) -> ("SMO"=w383:refnum<class "instrument.PPMS.lvclass">)
            n131 = call-dynamic "PPMS.getAll.vi"("error in (no error)"=w382, "instrument.PPMS in"=w383) -> ("error out"=w375:errorcluster, "getAll"=w376:T7, "instrument.PPMS out"=w379:refnum<class "instrument.PPMS.lvclass">)  [unwired: 7 in]
            n132 = call <userlib>:"setAllData.vi"("error in (no error)"=w375, "AllData"=w376, "Instrument in"=w379) -> ("error out"=w377:errorcluster, "Instrument out"=w378:refnum<class "instrument.PPMS.lvclass">)  [unwired: 7 in]
            n133 = Bundle By Name(cluster=w380, "SMO"=w378) -> (w381:T5)
            n134 = call <vilib>:"Add State(s) to Queue__jki_lib_state_machine.vi"("State(s) in (\"\")"=w386) -> ("States Out"=w385:string)  [unwired: 14 in]
          }
          frame "PPMS: Log" {
            n135 = Unbundle By Name(w400) -> ("SMO"=w394:refnum<class "instrument.PPMS.lvclass">)
            n136 = Unbundle By Name(w394) -> ("getAll"=w393:T7)
            n137 = call-dynamic "getAllsubset.vi"("error in (no error)"=w392, "getAll"=w393, "instrument.PPMS in"=w394) -> ("error out"=w391:errorcluster, "output cluster"=w387:variant, "instrument.PPMS out"=w389:refnum<class "instrument.PPMS.lvclass">)  [unwired: 6 in]
            "Log Data" <- w387
            n138 = call-dynamic "Get SMO Database Paths.vi"("error in (no error)"=w391, "instrument.PPMS in"=w389) -> ("error out"=w390:errorcluster, "Paths"=w395:string, "instrument.PPMS out"=w388:refnum<class "instrument.PPMS.lvclass">)  [unwired: 7 in]
            "Log Address" <- w395
            n139 = Empty String/Path?(string/path=w395) -> (empty?=w398:bool)
            n140 = Empty String/Path?(string/path=w387) -> (empty?=w397:bool)
            n141 = Or(x=w398, y=w397) -> (x .or. y?=w396:bool)
            n142 = case shown="False" w396 {
              tunnel: w395 -> [_ w413]
              tunnel: [w407 w412] -> w402
              tunnel: [w406 w411] -> w399
              tunnel: w390 -> [w406 w410]
              tunnel: w387 -> [_ w409]
              tunnel: w388 -> [w407 w408]
              frame True {
              }
              frame False {
                n143 = call <userlib>:"Instrument.logToDatabase.vi"("error in (no error)"=w410, "Data"=w409, "Paths"=w413, "Instrument"=w408) -> ("error out"=w411:errorcluster, "Instrument out"=w412:refnum<class "instrument.PPMS.lvclass">)  [unwired: 6 in]
              }
            }
            n144 = Bundle By Name(cluster=w400, "SMO"=w402) -> (w401:T5)
            n145 = call <vilib>:"Add State(s) to Queue__jki_lib_state_machine.vi"("State(s) in (\"\")"=w405) -> ("States Out"=w404:string)  [unwired: 14 in]
          }
          frame "PPMS: setAngle" {
            # "Template Separator\n(You can make a copy of, or modify, this frame)"
            n146 = Unbundle By Name(w419) -> ("SMO"=w418:refnum<class "instrument.PPMS.lvclass">, "MessageToProcess.Message.Data"=w417:variant)
            n147 = call "PPMS.setAngle.vi"("error in (no error)"=w416, "Data"=w417, "instrument.PPMS"=w418) -> ("error out"=w415:errorcluster, "instrument.PPMS out"=w414:refnum<class "instrument.PPMS.lvclass">)  [unwired: 7 in]
            n148 = Bundle By Name(cluster=w419, "SMO"=w414) -> (w420:T5)
            n149 = call <vilib>:"Add State(s) to Queue__jki_lib_state_machine.vi"("State(s) in (\"\")"=w423) -> ("States Out"=w422:string)  [unwired: 14 in]
          }
          frame "PPMS: setChamber" {
            # "Template Separator\n(You can make a copy of, or modify, this frame)"
            n150 = Unbundle By Name(w429) -> ("SMO"=w428:refnum<class "instrument.PPMS.lvclass">, "MessageToProcess.Message.Data"=w427:variant)
            n151 = call "PPMS.setChamber.vi"("error in (no error)"=w426, "Data"=w427, "instrument.PPMS"=w428) -> ("error out"=w425:errorcluster, "instrument.PPMS out"=w424:refnum<class "instrument.PPMS.lvclass">)  [unwired: 7 in]
            n152 = Bundle By Name(cluster=w429, "SMO"=w424) -> (w430:T5)
            n153 = call <vilib>:"Add State(s) to Queue__jki_lib_state_machine.vi"("State(s) in (\"\")"=w433) -> ("States Out"=w432:string)  [unwired: 14 in]
          }
          frame "PPMS: setMagnet" {
            # "Template Separator\n(You can make a copy of, or modify, this frame)"
            n154 = Unbundle By Name(w439) -> ("SMO"=w438:refnum<class "instrument.PPMS.lvclass">, "MessageToProcess.Message.Data"=w437:variant)
            n155 = call "PPMS.setMagnet.vi"("error in (no error)"=w436, "Data"=w437, "instrument.PPMS"=w438) -> ("error out"=w435:errorcluster, "instrument.PPMS out"=w434:refnum<class "instrument.PPMS.lvclass">)  [unwired: 7 in]
            n156 = Bundle By Name(cluster=w439, "SMO"=w434) -> (w440:T5)
            n157 = call <vilib>:"Add State(s) to Queue__jki_lib_state_machine.vi"("State(s) in (\"\")"=w443) -> ("States Out"=w442:string)  [unwired: 14 in]
          }
          frame "PPMS: setTemperature" {
            n158 = Unbundle By Name(w449) -> ("SMO"=w448:refnum<class "instrument.PPMS.lvclass">, "MessageToProcess.Message.Data"=w447:variant)
            n159 = call "PPMS.setTemperature.vi"("error in (no error)"=w446, "Data"=w447, "instrument.PPMS"=w448) -> ("error out"=w445:errorcluster, "instrument.PPMS out"=w444:refnum<class "instrument.PPMS.lvclass">)  [unwired: 7 in]
            n160 = Bundle By Name(cluster=w449, "SMO"=w444) -> (w450:T5)
            n161 = call <vilib>:"Add State(s) to Queue__jki_lib_state_machine.vi"("State(s) in (\"\")"=w453) -> ("States Out"=w452:string)  [unwired: 14 in]
          }
        }
      }
    }
    frame Error {
    }
  }
  n162 = call-parent "Process.vi"("error in"=w5, "Instrument"=w4) -> ("error out"=w2:errorcluster, "Instrument out"=→"instrument.PPMS out":refnum<class "instrument.PPMS.lvclass">)  [unwired: 8 in]
  n163 = Merge Errors(w2, w1) -> (→"error out":errorcluster)
